vi "GlobalSetGetPixelOfRoi.vi"() -> ()   [LabVIEW 2011]
panel:
  in  "Length Axial":dbl
  in  "Start Axial":dbl
  in  "Stepsize axial":dbl
  in  "ROI Y length":dbl
  in  "ROI Y Start":dbl
  in  "ROI X length":dbl
  in  "ROI X Start":dbl
  in  "ROI Pixel SizeX":dbl
  in  "ROI Pixel SizeY":dbl
  in  "ROI Pixel SizeZ":dbl
  in  "ROI Stack length":dbl
  in  "ROI Stack Start":dbl
  in  "Y length":dbl
  in  "Y Start":dbl
  in  "X length":dbl
  in  "X Start":dbl
  in  "Pixel SizeX":dbl
  in  "Pixel SizeY":dbl
  in  "Pixel SizeZ":dbl
  in  "Stack length":dbl
  in  "Stack Start":dbl
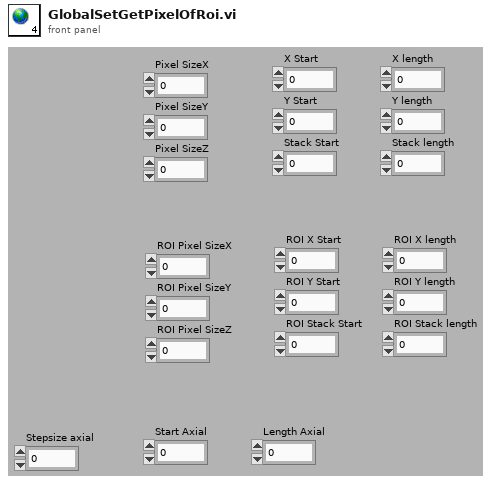
[diagram p1: front panel]
diagram:
